vi "PCP data gathering Loop.vi"(1 "Loop ID":T1=enum."Var Handling-From PCP", 11 "error in":errorcluster) -> ()   [LabVIEW 2011]
uses:
  Application Structure/Loop ID.ctl
  Action Analog Handler.ctl
  Common/Variable List Common Digital.ctl
  Common/Variable List Common Analog.ctl
  PCP interface/PCP return data types/RDd return.ctl
  PCP interface/PCP return data types/RA return Analog I.ctl
  PCP interface/PCP return data types/RP return digital IO.ctl
  Status Digitalish.ctl
  emi Lib/System 01/0 - General/App/Loop control 2/Private/_emi_ SMLoop start condition.vi
  emi Lib/System 01/0 - General/App/Loop control 2/Private/_emi_ SMLoop Error Check.vi
  emi Lib/Basic/0 - General/Error/emi_Is Error.vi
  emi Lib/System 01/0 - General/App/Loop control 2/Private/_emi_SMLoop Register new.vi
  emi Lib/System 01/0 - General/S&E reporting/emi_Send S&E Error message.vi
  emi Lib/Basic/0 - General/Error/emi_ Is Error state.vi
  emi Lib/System 01/0 - General/emi_Read System ID.vi
  emi Lib/System 01/0 - General/App/Loop control/Private/_emi_GFV Loop Linking.vi
  emi Lib/System 01/0 - General/App/Loop control/Private/_emi_GFV Loop Enable.vi
  emi Lib/System 01/0 - General/App/Loop control 2/Private/_emi_ SMLoop Restart.vi
  emi Lib/System 01/0 - General/App/Private/_emi_GFV App Close.vi
  emi Lib/System 01/0 - General/App/Loop control 2/Private/_emi_ SMLoop Restart Counter.vi
  emi Lib/System 01/0 - General/App/Loop control/Private/_emi_GFV Loop Running.vi
  emi Lib/System 01/0 - General/Private/_emi_GFV System ID.vi
  emi Lib/System 01/0 - General/S&E reporting/Private/_emi_S&E Q Generator.vi
  <vilib>/Utility/error.llb/Clear Errors.vi
  emi Lib/System 01/0 - General/App/Loop control/Private/_emi_GFV stop a loop so it can reset.vi
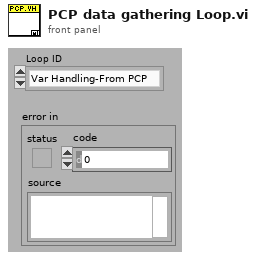
[diagram p1: front panel]
types:
  T1 = typedef "Loop ID.ctl" = enum16{"Main-QSM", "Main-Dialog", "Main-Ind Upd", "Main-Graph Upd", "Main-Debug", "Main-DebugW1", "Main-DebugW2", "Main-SE Handler", "Interface-PCP", "Interface-CANbus", "Interface-Modem", "Var Handling-Beat", "Var Handling-From PCP", "Var Handling-File storage", "Var Handling-From Simulator", "GUI-GrphW Mast", "GUI-GrphW Slav", "SIM-Tool W1", "SIM-Tool W2", "Alm-Sound", "LEIN-motor", "Tool data gatherer Qer", "Tool Data LEIN STAT2 dekoder", "Indicator Value Update", "Tool STAT2 dedicated reader", "Tool ID handler", "Detail View L1", "Detail View L2", "Main display enable view", "Sequence runner", "Voltage setpoint", "Resistance setpoint", "Stroker Wizard L1", "Stroker Wizard L2", "Alarm Handling", "Annotations Tip Strip", "Magna Interface", "Modem Status", "Var Handling - Modem Status", "Power interface detector"}
  T2 = typedef "Action Analog Handler.ctl" = enum16{"GET value", "GET Single Frequenzy", "GET All Values", "GET Waveform", "Get Numb Var", "SET Value", "START Buffer", "REG Variable", "BUF size(total antal sekund)", "PULS", "Get a Value at time", "Set initial waveform"}
  T3 = typedef "RDd return.ctl" = cluster{"AI":T4, "Depth counter(Raw)":i32, "General Ratemeter":dbl, "Digital ports":T5}
  T4 = typedef "RA return Analog I.ctl" = cluster{"HVPSU voltage output (AI 1)":dbl, "HVPSU current output (AI 2)":dbl, "PCP Motor voltage, head voltage (AI 3)":dbl, "PCP Cable resistance (AI 4)":dbl, "Cable tension (AI 5)":dbl, "CCL (AI 6)":dbl}
  T5 = typedef "RP return digital IO.ctl" = cluster{"DO -  HVPSU HV Off":bool, "DO -  HVPSU HV On":bool, "DI -  Unused 1":bool, "DO -  Local(T) / PC(F) mode":bool, "DI - Unused 2":bool, "DI - HVPSU HV On(T)":bool, "DI - PCP Local control(T)":bool, "DI - HVPSU On(T)":bool}
  T6 = typedef "Status Digitalish.ctl" = enum16{"NA", "False", "True"}
  T7 = typedef "_emi_ SMLoop sates.ctl" = enum16{"Init", "Standby", "Start", "Normal Operation", "Stop", "Error Handling", "End", "Post"}
  T8 = cluster{"Placeholder":bool, "PCP Ans Not":refnum<notifier>}
  T9 = typedef "Options  All pages and custom.ctl" = cluster{"P 1 (App)":T10, "P 2":T11, "P 3":T12, "P 4":T15, "P 5":T20, "P 6 (Err)":T21, "P 7 (Expert)":T22, "P 8 (Depth)":T24, "C 1":T25, "C 2":T26}
  T10 = typedef "Options Page 1 (App).ctl" = cluster{"Result files":path, "PCP Interface":string, "Tractor/Stroker Interface":string, "Tractor Interface":string, "Modem Status Interface":string, "Audible Alarm":bool, "Force alarm on Technical":bool, "Force alarm on HH":bool, "Force alarm on LL":bool, "Force alarm on H":bool, "Force alarm on L":bool}
  T11 = typedef "Options Page 2.ctl" = cluster{"Solenoid & Relay latching time":u16, "Tractor relay 1":dbl, "Tractor relay 2":dbl, "Tractor Solenoid limit":dbl}
  T12 = typedef "Options Page 3.ctl" = cluster{"Min resistance":dbl, "Max resistance":dbl, "Head voltage range":T13, "Max voltage jump":dbl, "Maximum resistance change":dbl, "Start Telemetry Voltage":dbl, "Start Telemetry Timeout":dbl, "Start Motor Voltage":dbl, "Stop Motor Voltage":dbl, "Pass Mode Warning Voltage":dbl, "Relay Switch Voltage":dbl, "Relay Status Loss Voltage":dbl, "Samples to average":i32, "PSU type DO NOT USE":T14, "Magna OVP":dbl, "Magna Current Limit":dbl}
  T13 = typedef "PCP type List.ctl" = enum16{"0 - 350V", "0 - 450V", "0 - 600V"}
  T14 = typedef "PSU Type.ctl" = enum16{"Unipower", "Magna 8.3A", "Magna 12A", "None"}
  T15 = typedef "Options Page 4.ctl" = cluster{"Solenoid & Relay latching time":u16, "Stroker relay 1":dbl, "Stroker Relay 2":dbl, "Stroker Solenoid limit":dbl, "Force det.":T16, "Stroke force lim.":dbl, "Anchor Enabled Pressure":dbl, "Tacometer puls":dbl, "Default anchor behavior":T17, "Default stroker behavior":T18, "Default stroker force limit (tonne)":dbl, "Slips Size":T19}
  T16 = typedef "Stroke force selector.ctl" = enum16{"Stroke in = node 1", "Strok out = node 1"}
  T17 = typedef "Default anchor behavior.ctl" = enum16{"Do nothing", "Set Anchor", "Release Anchor"}
  T18 = typedef "Default stroker behavior.ctl" = enum16{"Do nothing", "Stop", "Go Out", "Go In"}
  T19 = typedef "Slips Type Radio.ctl" = enum32{"No Selection", "338 MRS", "3,9 MRS"}
  T20 = typedef "Options Page 5.ctl" = cluster{"Solenoid & Relay latching time":u16, "Driller relay 1":dbl, "Driller Relay 2":dbl, "Driller  Solenoid limit":dbl}
  T21 = typedef "Options Page 6 (Err).ctl" = cluster{"Error and event files":path}
  T22 = typedef "Options Page 7 (Expert).ctl" = cluster{"Show Debug":bool, "Log debug messages":bool, "Additional debug messages":bool, "Start Beagle with Simulator data":bool, "Workshop mode":bool, "Modem baud":u16, "enumCANCOM":bool, "Modem sim":T23, "Telemetry Timeout Disable":i32, "Buffer size":i32, "Upd regular data":bool, "Cable comp":cluster{"VMOD1 Voltage(V)":dbl, "VMOD2 Voltage(V)":dbl}}
  T23 = typedef "Modem simulation setup.ctl" = cluster{"Modem dealay sim":bool, "Sim baud Tx":u16, "Bit Error fraction Tx":dbl, "Sim baud Rx":u16, "Bit Error fraction Rx":dbl}
  T24 = typedef "Options Page 8 (Depth).ctl" = cluster{"Winch Spool Circumference":dbl, "Winch Pulses per Revolution":dbl, "Current Depth":dbl}
  T25 = typedef "Options Custom 1.ctl" = cluster{"Depth Updated":bool, "Depth Offset":dbl}
  T26 = typedef "Options Custom 2.ctl" = cluster{"Placeholder":bool}
  T27 = typedef "Fixed Analog Channel Definition.ctl" = cluster{"ID":u16, "Name":string, "Quantity":T28, "Unit":string, "Maximum upd":T29, "Comment":string, "Help file Name":string, "Help file Section ":string, "Category":T30, "User adjustable Scaling":bool, "Default Scaling":T31, "Default Unit":i32, "Classification":T32}
  T28 = typedef "Quantity enum.ctl" = enum16{"NA", "Acceleration", "Angle", "Current", "Force", "Distance", "Pressure", "Resistance", "Rotational Speed", "Speed", "Temperature", "Tension", "Torque", "Voltage", "Weight"}
  T29 = typedef "Update frequensies.ctl" = enum16{"2 Hz", "1 Hz", "0.1 Hz"}
  T30 = typedef "Channel catagory Enum.ctl" = enum16{"No Category", "Power", "Temperature", "Pressure"}
  T31 = typedef "Scaling.ctl" = cluster{"Gain":dbl, "Offset":dbl}
  T32 = typedef "Channel Classification Enum.ctl" = enum16{"Basic", "Advanced", "Expert", "Unused"}
  T33 = typedef "Fixed Digital Channel Definition.ctl" = cluster{"ID":u16, "Name":string, "NA Text":string, "Off Text":string, "On Text":string, "Maximum upd":T29, "Comment":string, "Help file Name":string, "Help file Section ":string, "Catagory":T30, "In use":bool}
  T34 = typedef "Variable List Common Digital.ctl" = enum16{"PCP Connected", "PCP PC Control", "HV PSU connected", "HV PSU HV Active", "Modem Connected", "Tool Connected", "CanBus interface"}
  T35 = typedef "Variable List Common Analog.ctl" = enum16{"HVPSU Head Voltage", "HVPSU TS Voltage", "HVPSU Current", "PCP Cable Resistance", "Winch Depth", "Winch Line Speed", "Winch Wire Tension"}
  T36 = typedef "PCP Command Return.ctl" = cluster{"Action":T37, "Data in return":variant}
  T37 = typedef "PCP Commands.ctl" = enum16{"do not use HE - Help", "RDd - Most used inputs", "RA - All analog inputs", "RE n Reset DO n", "SE n Set DO n", "RP - Get digital inputs", "VA d Set AO A  Motor Volt", "VB d Set AO B  Cable Resistance", "VEr - Get Version", "DYp - Depth counter", "DR - Reset Depth Counter", "DS n Set Depth options(0-3)", "do not use ME - Manual mode enabled", "MD - Manual mode disabled", "ID - Get ID(2001)", "TS - Get Timestamp", "TO d(s)  Set timeout", "do not use LO n Start Loop Mode(1,2)", "AL n RD&LO variation", "ST - Stop Loop Mode"}
  T38 = typedef "Connected Satus Bool.ctl" = bool
  T39 = typedef "Active Status Bool.ctl" = bool
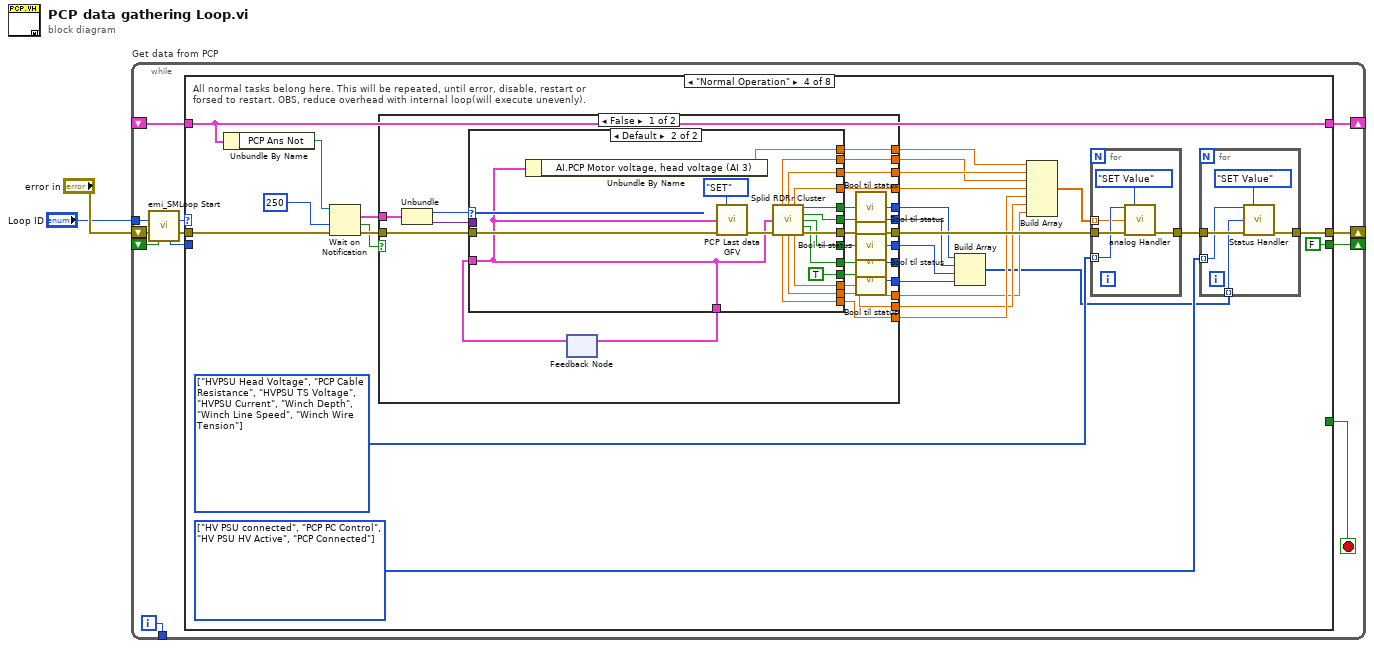
[diagram p0: block diagram]
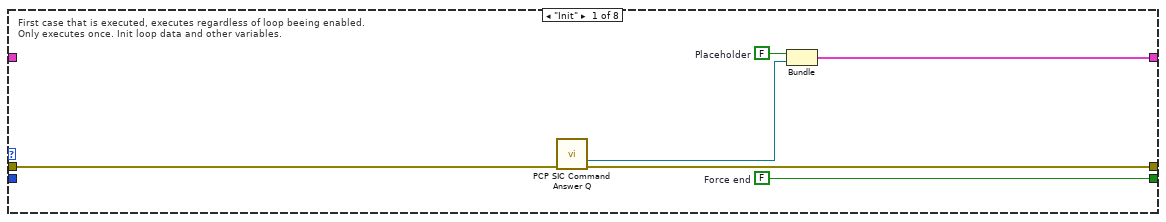
[diagram p2: hidden frame]
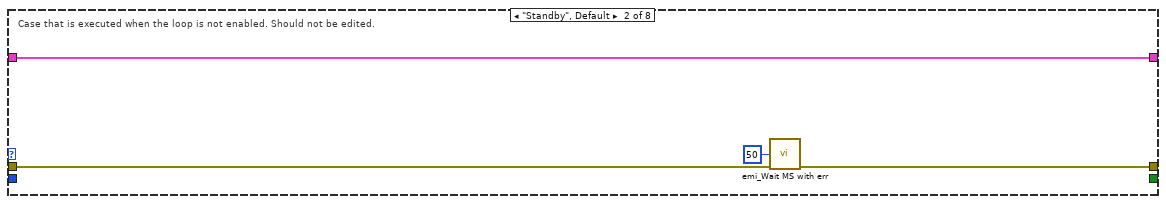
[diagram p3: hidden frame]
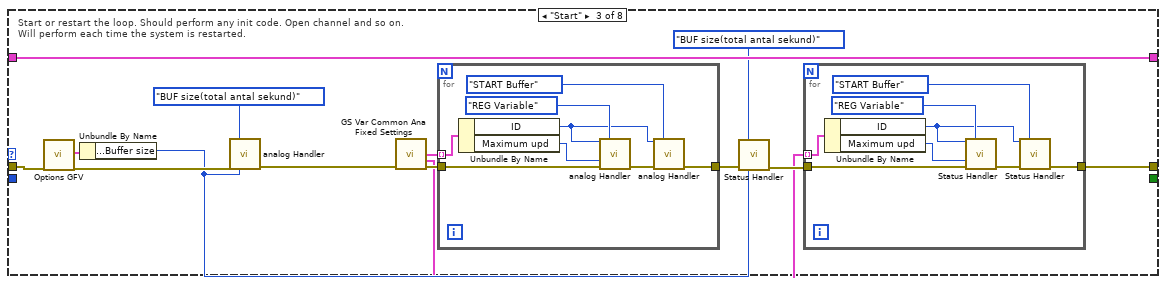
[diagram p4: hidden frame]
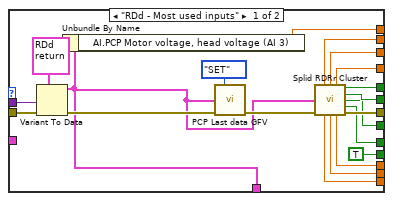
[diagram p5: hidden frame]
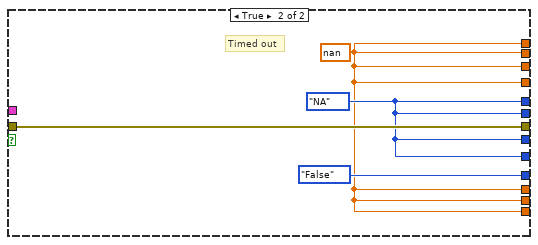
[diagram p6: hidden frame]
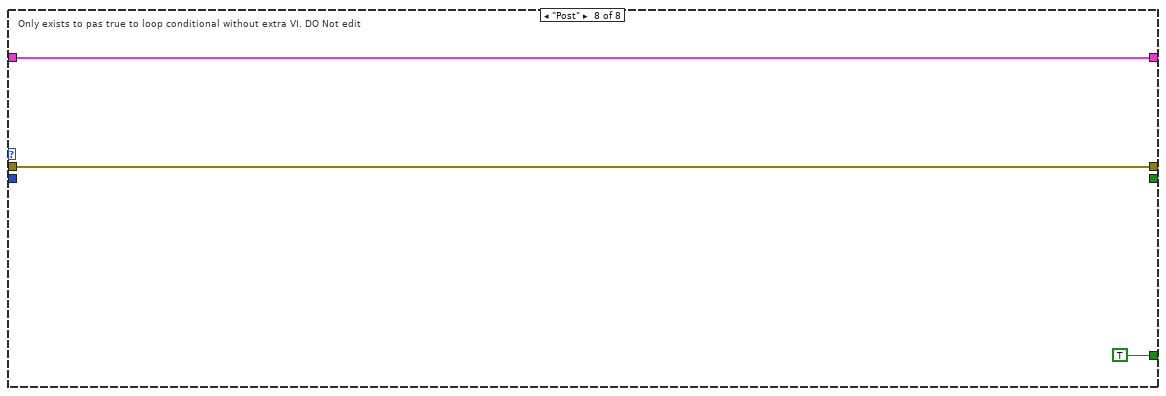
[diagram p10: hidden frame]
diagram:
  n1 = while "Get data from PCP" {
    shift-right: [w14] -> _
    shift-left: _ -> [w11]
    tunnel: [w12] -> _
    shift-right: [w10] -> _
    shift-left: _ -> [w5]
    tunnel: "Loop ID" -> [w6]
    shift-right: [w3] -> _
    shift-left: "error in" -> [w9]
    i -> [w12]
    stop <- w13 stop-if-true
    n2 = call "emi_SMLoop Start.vi"("Loop ID"=w6, "error in (no error)"=w9, "Force Stop(F)"=w5) -> ("Loop command"=w7:T7, "error out"=w8:errorcluster, "Loop ID out"=w4:i32)  [unwired: 10 in]
    n3 = case shown="\"Normal Operation\"" w7 {
      tunnel: [w20 w21 w38 w79 w156 w159 w160 w163] -> w14
      tunnel: [_ _ _ _ _ _ _ TRUE] -> w13
      tunnel: w8 -> [w17 w23 w36 w80 w157 w158 w161 w164]
      tunnel: [w16 w22 w26 w77 w157 w158 w161 w164] -> w3
      tunnel: w11 -> [_ w21 w38 w79 w156 w159 w160 w163]
      tunnel: [w18 _ _ FALSE ("Force End") _ _ _ _] -> w10
      tunnel: w4 -> [_ _ _ _ _ _ _ _]
      frame "Init" {
        w18 = FALSE  # Force end
        w19 = FALSE  # Placeholder
        # "First case that is executed, executes regardless of loop beeing enabled.\nOnly executes once. Init loop data and other variables."
        n4 = call "PCP SIC Command Answer Q.vi"("error in (no error)"=w17) -> ("PCP Ans Not"=w15:refnum<notifier>, "error out"=w16:errorcluster)  [unwired: 12 in, 1 out]
        n5 = Bundle("Placeholder"=w19, "PCP Ans Not"=w15) -> (w20:T8)  [unwired: 1 in]
      }
      frame "Standby", Default {
        # "Case that is executed when the loop is not enabled. Should not be edited."
        n6 = call "emi_Wait MS with err.vi"("milliseconds to wait(0)"=u32 50, "error in (no error)"=w23) -> ("error out"=w22:errorcluster)  [unwired: 13 in]
      }
      frame "Start" {
        # "Start or restart the loop. Should perform any init code. Open channel and so on. \nWill perform each time the system is restarted."
        n7 = call "Options GFV.vi"("error in (no error)"=w36) -> ("Options"=w34:T9, "error out"=w35:errorcluster)  [unwired: 16 in, 1 out]
        n8 = Unbundle By Name(w34) -> ("P 7 (Expert).Buffer size"=w29:i32)
        n9 = call "analog Handler.vi"("Action"=Action_Analog_Handler."BUF size(total antal sekund)" ("Action(GET)"), "error in (no error)"=w35, "Start tid / buf size"=w29) -> ("error out"=w33:errorcluster)  [unwired: 7 in, 5 out]
        n10 = call "GS Var Common Ana Fixed Settings.vi"("error in (no error)"=w33) -> ("Common Analog Var Fixed out"=w31:T27[], "Common Digital var Fixed"=w25:T33[], "error out"=w32:errorcluster)  [unwired: 12 in]
        n11 = for {
          tunnel: [w49] -> w30
          tunnel: w32 -> [w54]
          tunnel: w31 -> [w53] mode=indexing
          n12 = Unbundle By Name(w53) -> ("ID"=w48:u16, "Maximum upd"=w52:T29)
          n13 = call "analog Handler.vi"("Variable Index"=w48, "Action"=Action_Analog_Handler."REG Variable" ("Action(GET)"), "Upd freq"=w52, "error in (no error)"=w54) -> ("error out"=w50:errorcluster)  [unwired: 6 in, 5 out]
          n14 = call "analog Handler.vi"("Variable Index"=w48, "Action"=Action_Analog_Handler."START Buffer" ("Action(GET)"), "error in (no error)"=w50) -> ("error out"=w49:errorcluster)  [unwired: 7 in, 5 out]
        }
        n15 = call "Status Handler.vi"("Action"=Action_Analog_Handler."BUF size(total antal sekund)", "error in (no error)"=w30, "Start tid(buff size"=w29) -> ("error out"=w27:errorcluster)  [unwired: 8 in, 4 out]
        n16 = for {
          tunnel: [w41] -> w26
          tunnel: w27 -> [w46]
          tunnel: w25 -> [w45] mode=indexing
          n17 = Unbundle By Name(w45) -> ("ID"=w40:u16, "Maximum upd"=w44:T29)
          n18 = call "Status Handler.vi"("Variable Index"=w40, "Action"=Action_Analog_Handler."REG Variable" ("Action(GET)"), "Upd freq"=w44, "error in (no error)"=w46) -> ("error out"=w42:errorcluster)  [unwired: 7 in, 4 out]
          n19 = call "Status Handler.vi"("Variable Index"=w40, "Action"=Action_Analog_Handler."START Buffer" ("Action(GET)"), "error in (no error)"=w42) -> ("error out"=w41:errorcluster)  [unwired: 8 in, 4 out]
        }
      }
      frame "Normal Operation" {
        w63 = T34[] [enum."HV PSU connected", enum."PCP PC Control", enum."HV PSU HV Active", enum."PCP Connected"] items=["PCP Connected", "PCP PC Control", "HV PSU connected", "HV PSU HV Active", "Modem Connected", "Tool Connected", "CanBus interface"]
        w65 = T35[] [enum."HVPSU Head Voltage", enum."PCP Cable Resistance", enum."HVPSU TS Voltage", enum."HVPSU Current", enum."Winch Depth", enum."Winch Line Speed", enum."Winch Wire Tension"] items=["HVPSU Head Voltage", "HVPSU TS Voltage", "HVPSU Current", "PCP Cable Resistance", "Winch Depth", "Winch Line Speed", "Winch Wire Tension"]
        # "All normal tasks belong here. This will be repeated, until error, disable, restart or\nforsed to restart. OBS, reduce overhead with internal loop(will execute unevenly)."
        n20 = Unbundle By Name(w79) -> ("PCP Ans Not"=w75:refnum<notifier>)
        n21 = Wait on Notification(notifier=w75, timeout in ms (-1)=250, error in (no error)=w80) -> (notification=w74:T36, timed out?=w72:bool, error out=w73:errorcluster)  [unwired: 1 in, 1 out]
        n22 = case shown="False" w72 {
          tunnel: w74 -> [w114 _]
          tunnel: [w113 w155] -> w71
          tunnel: w73 -> [w112 w155]
          tunnel: [w109 w152] -> w56
          tunnel: [w108 w152] -> w57
          tunnel: [w107 w152] -> w66
          tunnel: [w106 w152] -> w69
          tunnel: [w105 w152] -> w70
          tunnel: [w92 w154] -> w62
          tunnel: [w94 w154] -> w58
          tunnel: [w96 w154] -> w61
          tunnel: [w98 w154] -> _
          tunnel: [w100 Status_Digitalish."False" ("Status")] -> w60
          tunnel: [w102 w152] -> w68
          tunnel: [w91 w152] -> w55
          frame False {
            n23 = Unbundle(w114) -> ("Action"=w111:T37, "Data in return"=w110:variant)
            n24 = feedback #1() -> (w103:T3)  [unwired: 1 in]
            n25 = case shown="Default" w111 {
              tunnel: [w131 w151] -> w113
              tunnel: w112 -> [w134 w138]
              tunnel: w110 -> [w133 _]
              tunnel: [w130 w150] -> w109
              tunnel: [w117 w149] -> w108
              tunnel: [w129 w148] -> w107
              tunnel: [w128 w147] -> w106
              tunnel: [w127 w146] -> w105
              tunnel: [w126 w145] -> w93
              tunnel: [w125 w144] -> w95
              tunnel: [w124 w143] -> w97
              tunnel: [w123 w142] -> w99
              tunnel: [TRUE TRUE] -> w101
              tunnel: [w115 w136] -> w104
              tunnel: w103 -> [_ w136]
              tunnel: [w121 w140] -> w102
              tunnel: [w116 w135] -> w91
              frame "RDd - Most used inputs" {
                n26 = Variant To Data(error in=w134, type=T3 {"AI"={"HVPSU voltage output (AI 1)"=0.0, "HVPSU current output (AI 2)"=0.0, "PCP Motor voltage, head voltage (AI 3)"=0.0, "PCP Cable resistance (AI 4)"=0.0, "Cable tension (AI 5)"=0.0, "CCL (AI 6)"=0.0}, "Depth counter(Raw)"=0, "General Ratemeter"=0.0, "Digital ports"={"DO -  HVPSU HV Off"=FALSE, "DO -  HVPSU HV On"=FALSE, "DI -  Unused 1"=FALSE, "DO -  Local(T) / PC(F) mode"=FALSE, "DI - Unused 2"=FALSE, "DI - HVPSU HV On(T)"=FALSE, "DI - PCP Local control(T)"=FALSE, "DI - HVPSU On(T)"=FALSE}} ("Periodic data"), Variant=w133) -> (data=w115:T3, error out=w120:errorcluster)
                n27 = Unbundle By Name(w115) -> ("AI.PCP Motor voltage, head voltage (AI 3)"=w116:dbl)
                n28 = call "PCP Last data GFV.vi"("Action(GET)"=enum16{"GET", "SET"}."SET", "PCP Data in"=w115, "error in (no error)"=w120) -> ("error out"=w119:errorcluster)  [unwired: 10 in, 2 out]
                n29 = call "Splid RDRr Cluster.vi"("Periodic data"=w115, "Error in"=w119) -> ("Common TS.V"=w130:dbl, "Common Wire.R"=w117:dbl, "Common Wire.I"=w129:dbl, "Connected Indicator PSU"=w126:T38, "Connected Indicator PPC PC Cont"=w125:T39, "Connected Indicator PSU HV On"=w124:T39, "Connected Indicator PSU Winch Moving"=w123:T39, "Common Wire.Len"=w127:dbl, "Common Wire.Speed"=w128:dbl, "Common Wire.Tension"=w121:dbl, "error out"=w131:errorcluster)  [unwired: 3 in]
              }
              frame Default {
                n30 = Unbundle By Name(w136) -> ("AI.PCP Motor voltage, head voltage (AI 3)"=w135:dbl)
                n31 = call "PCP Last data GFV.vi"("Action(GET)"=enum16{"GET", "SET"}."SET", "PCP Data in"=w136, "error in (no error)"=w138) -> ("error out"=w137:errorcluster)  [unwired: 10 in, 2 out]
                n32 = call "Splid RDRr Cluster.vi"("Periodic data"=w136, "Error in"=w137) -> ("Common TS.V"=w150:dbl, "Common Wire.R"=w149:dbl, "Common Wire.I"=w148:dbl, "Connected Indicator PSU"=w145:T38, "Connected Indicator PPC PC Cont"=w144:T39, "Connected Indicator PSU HV On"=w143:T39, "Connected Indicator PSU Winch Moving"=w142:T39, "Common Wire.Len"=w146:dbl, "Common Wire.Speed"=w147:dbl, "Common Wire.Tension"=w140:dbl, "error out"=w151:errorcluster)  [unwired: 3 in]
              }
            }
            n33 = feedback-in #1(w104) -> ()
            n34 = call "Bool til status.vi"("Boolean"=w93) -> ("Status"=w92:T6)  [unwired: 8 in]
            n35 = call "Bool til status.vi"("Boolean"=w95) -> ("Status"=w94:T6)  [unwired: 8 in]
            n36 = call "Bool til status.vi"("Boolean"=w97) -> ("Status"=w96:T6)  [unwired: 8 in]
            n37 = call "Bool til status.vi"("Boolean"=w99) -> ("Status"=w98:T6)  [unwired: 8 in]
            n38 = call "Bool til status.vi"("Boolean"=w101) -> ("Status"=w100:T6)  [unwired: 8 in]
          }
          frame True {
            w154 = Status_Digitalish."NA" ("Status")
            w152 = nan ("Common TS.V")
            # "Timed out"
          }
        }
        n39 = Build Array(w62, w58, w61, w60) -> (w59:T6[])
        n40 = Build Array(w55, w57, w56, w66, w70, w69, w68) -> (w67:dbl[])
        n41 = for {
          tunnel: w71 -> [w90]
          tunnel: [w89] -> w64
          tunnel: w65 -> [w88] mode=indexing
          tunnel: w67 -> [w86] mode=indexing
          n42 = call "analog Handler.vi"("Variable Index"=w88, "Action"=Action_Analog_Handler."SET Value" ("Action(GET)"), "Value"=w86, "error in (no error)"=w90) -> ("error out"=w89:errorcluster)  [unwired: 6 in, 5 out]
        }
        n43 = for {
          tunnel: w64 -> [w85]
          tunnel: [w84] -> w77
          tunnel: w63 -> [w82] mode=indexing
          tunnel: w59 -> [w81] mode=indexing
          n44 = call "Status Handler.vi"("Variable Index"=w82, "Action"=Action_Analog_Handler."SET Value" ("Action(GET)"), "Value"=w81, "error in (no error)"=w85) -> ("error out"=w84:errorcluster)  [unwired: 7 in, 4 out]
        }
      }
      frame "Stop" {
        # "Stop the loop. May be restarted later. Close interfaces and the like"
      }
      frame "Error Handling" {
        # "Loop automaticaly returns here after error is found. If error is cleared, Loop wil continue\nas normal(if was operative when error."
      }
      frame "End" {
        # "Only executes at application end has. Should performa any action the loop needs to finnish. \nExecutes only once."
      }
      frame "Post" {
        # "Only exists to pas true to loop conditional without extra VI. DO Not edit"
      }
    }
  }
